vi "Set Speed.vi"(8 "error in (no error)":errorcluster, 10 "speed (ml/min)":dbl min=0.0 max=999.99 format="%06.2f", 11 "SSI PR Settings":T1) -> (0 "error out":errorcluster, 1 "Connection Error":bool, 3 "SSI PR Settings":T1)   [LabVIEW 2018, in "SSI PR Pump.lvlib"]
uses:
  SSI PR Pump.lvlib
  SSI PR Settings Cluster.ctl
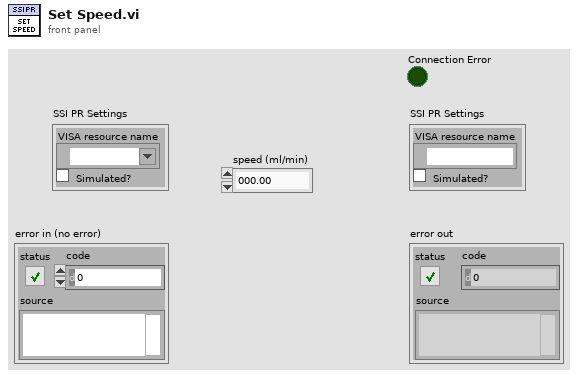
[diagram p1: front panel]
types:
  T1 = typedef "SSI PR Pump.lvlib/SSI PR Settings Cluster.ctl" = cluster{"VISA resource name":refnum<visa-resource-name>, "Simulated?":bool}
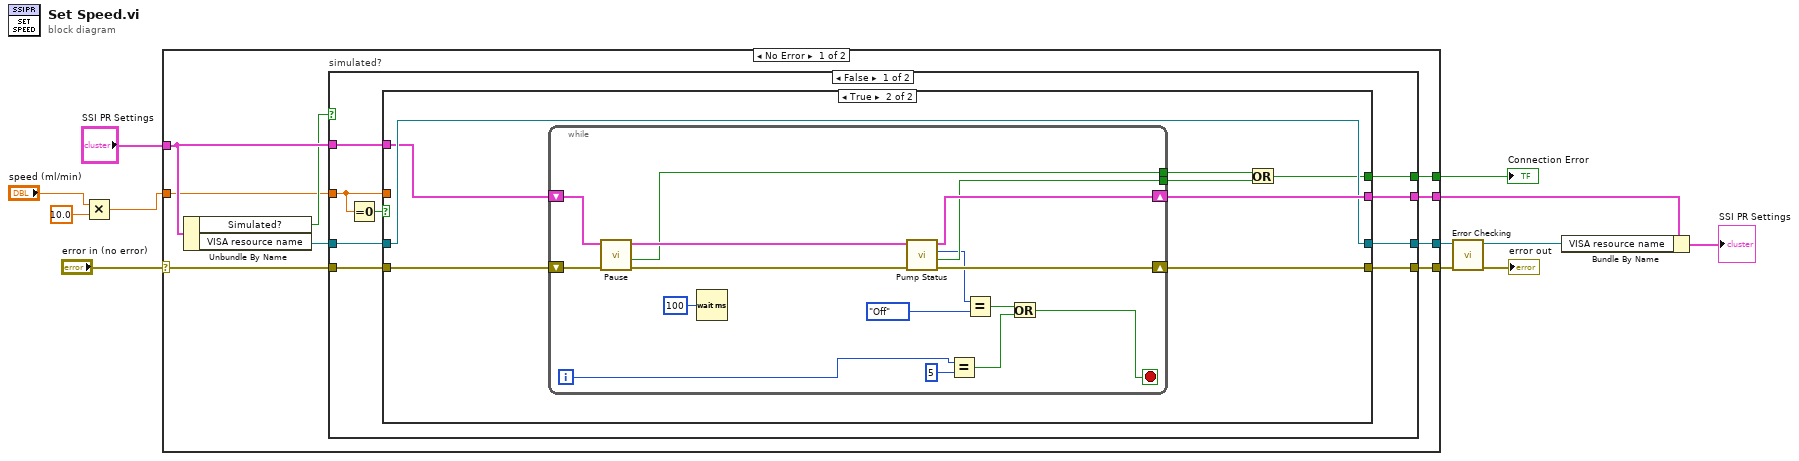
[diagram p0: block diagram]
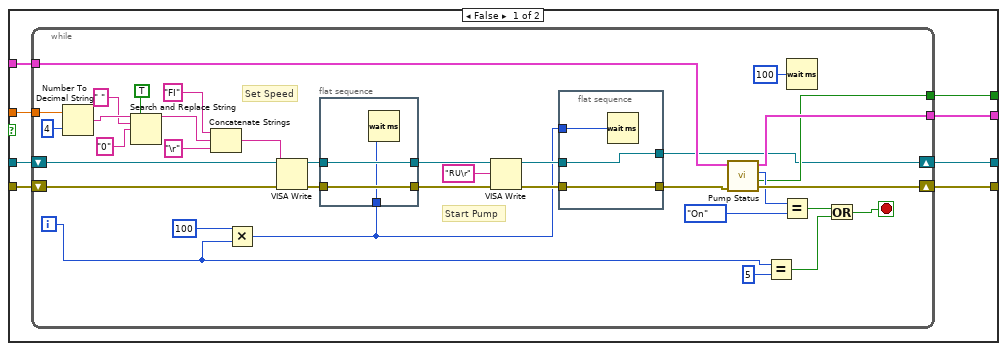
[diagram p2: hidden frame]
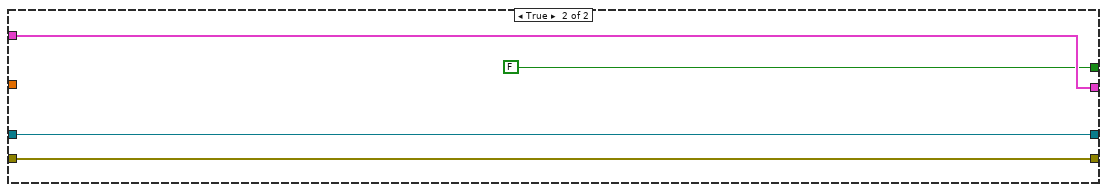
[diagram p3: hidden frame]
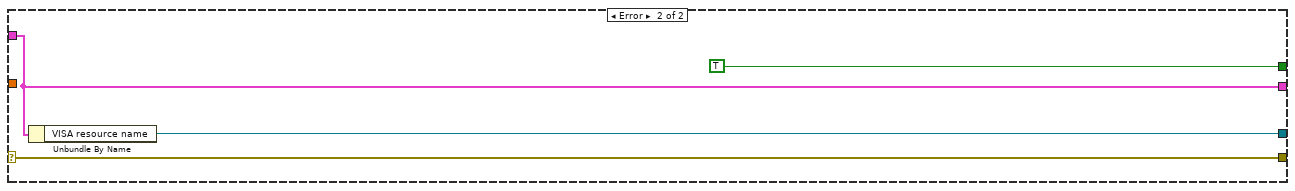
[diagram p4: hidden frame]
diagram:
  n1 = Multiply(x="speed (ml/min)", y=10.0) -> (x*y=w1:dbl)
  n2 = case shown="No Error" "error in (no error)" {
    selector: "error in (no error)" -> [w21 w111]
    tunnel: [w17 w110] -> w8
    tunnel: "SSI PR Settings" -> [w18 w110]
    tunnel: [w20 w109] -> w12
    tunnel: [w19 w111] -> w11
    tunnel: [w16 TRUE ("Connection Error")] -> w4
    tunnel: w1 -> [w13 _]
    frame No Error {
      n3 = Unbundle By Name(w18) -> ("Simulated?"=w15:bool, "VISA resource name"=w14:refnum<visa-resource-name>)
      n4 = case "simulated?" shown="False" w15 {
        tunnel: [w28 w107] -> w20
        tunnel: w14 -> [w30 w107]
        tunnel: w21 -> [w29 w106]
        tunnel: [w27 w106] -> w19
        tunnel: w18 -> [w26 w105]
        tunnel: [w25 w105] -> w17
        tunnel: [w24 FALSE ("Connection Error")] -> w16
        tunnel: w13 -> [w22 _]
        frame False {
          n5 = Equal To 0?(x=w22) -> (x = 0?=w23:bool)
          n6 = case shown="True" w23 {
            tunnel: w30 -> [w38 w85]
            tunnel: w29 -> [w37 w83]
            tunnel: [w36 w85] -> w28
            tunnel: [w35 w87] -> w27
            tunnel: w26 -> [w34 w84]
            tunnel: [w33 w86] -> w25
            tunnel: [w32 w80] -> w24
            tunnel: w22 -> [w31 _]
            frame False {
              n7 = while {
                shift-right: [w49] -> w36
                shift-left: w38 -> [w64]
                shift-right: [w70] -> w35
                shift-left: w37 -> [w62]
                tunnel: w34 -> [w68]
                tunnel: [w69] -> w33
                tunnel: [w61] -> w32
                tunnel: w31 -> [w60]
                i -> [w41]
                stop <- w42 stop-if-true
                # "Set Speed"
                # "Start Pump"
                n8 = Number To Decimal String(number=w60, width (-)=i16 4) -> (decimal integer string=w58:string)
                n9 = Search and Replace String(replace all?=TRUE ("replace all? (F)"), input string=w58, search string=" ", replace string="0" ("replace string (\"\")")) -> (result string=w57:string)  [unwired: 4 in, 3 out]
                n10 = Concatenate Strings("FI" ("string"), w57, "\r" ("string")) -> (w65:string)
                n11 = Multiply(x=u32 100 ("milliseconds to wait"), y=w41) -> (x*y=w39:u32)
                n12 = VISA Write(VISA resource name=w64, write buffer=w65, error in (no error)=w62) -> (VISA resource name out=w52:refnum<visa-resource-name>, error out=w50:errorcluster)  [unwired: 1 out]
                n13 = flat-sequence {
                  tunnel: [w79] -> w53
                  tunnel: w52 -> [w79]
                  tunnel: [w78] -> w51
                  tunnel: w50 -> [w78]
                  tunnel: w39 -> [w77]
                  frame #0 {
                    n14 = Wait (ms)(milliseconds to wait=w77) -> ()  [unwired: 1 out]
                  }
                }
                n15 = VISA Write(VISA resource name=w53, write buffer="RU\r" ("string"), error in (no error)=w51) -> (VISA resource name out=w48:refnum<visa-resource-name>, error out=w46:errorcluster)  [unwired: 1 out]
                n16 = flat-sequence {
                  tunnel: [w76] -> w49
                  tunnel: w48 -> [w76]
                  tunnel: [w75] -> w47
                  tunnel: w46 -> [w75]
                  tunnel: w39 -> [w74]
                  frame #0 {
                    n17 = Wait (ms)(milliseconds to wait=w74) -> ()  [unwired: 1 out]
                  }
                }
                n18 = call "Pump Status.vi"("error in (no error)"=w47, "SSI PR Settings"=w68) -> ("error out"=w70:errorcluster, "Connection Error"=w61:bool, "Pump On?"=w67:enum16{"Off", "On", "Not Initialized"}, "SSI PR Settings"=w69:T1)  [unwired: 4 in, 2 out]
                n19 = Equal?(x=w41, y=5) -> (x = y?=w43:bool)
                n20 = Equal?(x=w67, y=enum16{"Off", "On", "Not Initialized"}."On") -> (x = y?=w44:bool)
                n21 = Wait (ms)(milliseconds to wait=u32 100) -> ()  [unwired: 1 out]
                n22 = Or(x=w44, y=w43) -> (x .or. y?=w42:bool)
              }
            }
            frame True {
              n23 = while {
                tunnel: [w97] -> w82
                tunnel: [w96] -> w81
                shift-right: [w102] -> w86
                shift-left: w84 -> [w101]
                shift-right: [w103] -> w87
                shift-left: w83 -> [w100]
                i -> [w89]
                stop <- w90 stop-if-true
                n24 = call "Pause.vi"("error in (no error)"=w100, "SSI PR Settings"=w101) -> ("error out"=w99:errorcluster, "Connection Error"=w96:bool, "SSI PR Settings"=w98:T1)  [unwired: 6 in]
                n25 = Wait (ms)(milliseconds to wait=u32 100) -> ()  [unwired: 1 out]
                n26 = call "Pump Status.vi"("error in (no error)"=w99, "SSI PR Settings"=w98) -> ("error out"=w103:errorcluster, "Connection Error"=w97:bool, "Pump On?"=w92:enum16{"Off", "On", "Not Initialized"}, "SSI PR Settings"=w102:T1)  [unwired: 4 in, 2 out]
                n27 = Equal?(x=w89, y=5) -> (x = y?=w93:bool)
                n28 = Equal?(x=w92, y=enum16{"Off", "On", "Not Initialized"}."Off") -> (x = y?=w91:bool)
                n29 = Or(x=w91, y=w93) -> (x .or. y?=w90:bool)
              }
              n30 = Or(x=w81, y=w82) -> (x .or. y?=w80:bool)
            }
          }
        }
        frame True {
        }
      }
    }
    frame Error {
      n31 = Unbundle By Name(w110) -> ("VISA resource name"=w109:refnum<visa-resource-name>)
    }
  }
  "Connection Error" <- w4
  n32 = call "Error Checking.vi"("error in (no error)"=w11, "VISA resource name"=w12) -> ("error out"=→"error out":errorcluster, "VISA resource name"=w10:refnum<visa-resource-name>)  [unwired: 7 in, 1 out]
  n33 = Bundle By Name(cluster=w8, "VISA resource name"=w10) -> (→"SSI PR Settings":T1)
